vi "find_parameters.vi"(10 "script input":string) -> (0 "Parameter Array":string[](array[string]), 1 "plotnames":string, 2 "parameter string":string, 3 "command":string, 4 "number of parameters":u8)   [LabVIEW 2017]
doc: "splits the command, parameters and plotname from the input string.\n\ncommand syntax:\n\ncommand(param1;param2;...)->plot_name"
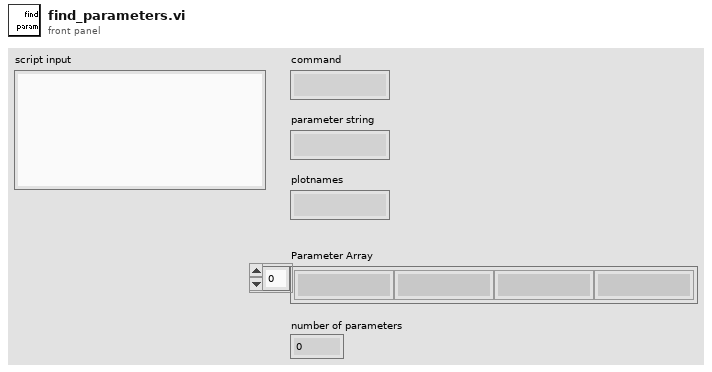
[diagram p1: front panel]
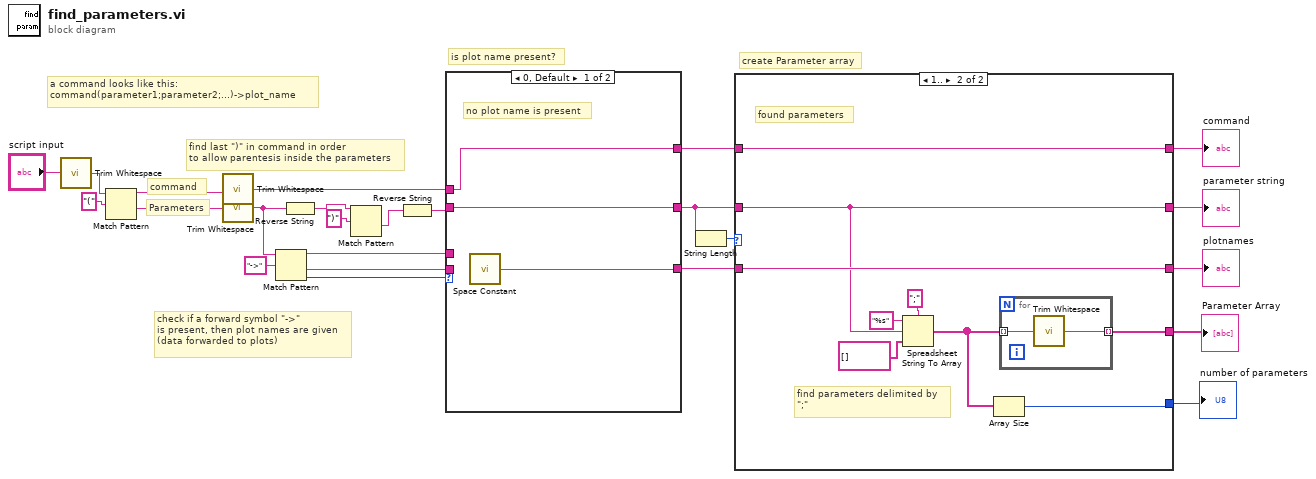
[diagram p0: block diagram]
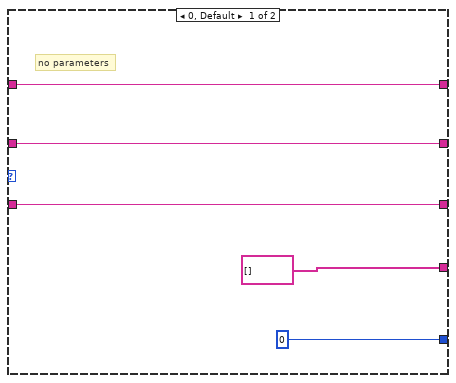
[diagram p2: hidden frame]
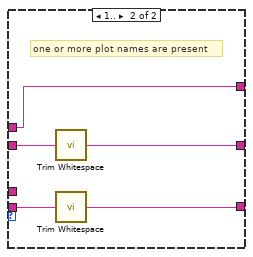
[diagram p3: hidden frame]
diagram:
  # "find last \")\" in command in order\nto allow parentesis inside the parameters"
  # "a command looks like this:\ncommand(parameter1;parameter2;...)->plot_name"
  # "is plot name present?"
  # "create Parameter array"
  # "Parameters"
  # "check if a forward symbol \"->\"\nis present, then plot names are given\n(data forwarded to plots)"
  # "command"
  n1 = call <vilib>:"Trim Whitespace.vi"("string"="script input") -> ("trimmed string"=w21:string)  [unwired: 1 in]
  n2 = Match Pattern(string=w21, regular expression="(") -> (before substring=w24:string, after substring=w23:string)  [unwired: 1 in, 2 out]
  n3 = call <vilib>:"Trim Whitespace.vi"("string"=w24) -> ("trimmed string"=w20:string)  [unwired: 1 in]
  n4 = call <vilib>:"Trim Whitespace.vi"("string"=w23) -> ("trimmed string"=w4:string)  [unwired: 1 in]
  n5 = Match Pattern(string=w4, regular expression="->") -> (before substring=w17:string, after substring=w16:string, offset past match=w18:i32)  [unwired: 1 in, 1 out]
  n6 = Reverse String(1:w4) -> (0:w3:string)
  n7 = Match Pattern(string=w3, regular expression=")") -> (after substring=w2:string)  [unwired: 1 in, 3 out]
  n8 = Reverse String(1:w2) -> (0:w1:string)
  n9 = case shown="0, Default" w18 {
    tunnel: w20 -> [w27 w32]
    tunnel: w1 -> [w25 w28]
    tunnel: [w27 w32] -> w13
    tunnel: [w25 w31] -> w10
    tunnel: [w26 w29] -> w12
    tunnel: w17 -> [_ _]
    tunnel: w16 -> [_ w30]
    frame 0, Default {
      # "no plot name is present"
      n10 = call <vilib>:"Space Constant.vi"() -> ("String"=w26:string)
    }
    frame 1.. {
      # "one or more plot names are present"
      n11 = call <vilib>:"Trim Whitespace.vi"("string"=w28) -> ("trimmed string"=w31:string)  [unwired: 1 in]
      n12 = call <vilib>:"Trim Whitespace.vi"("string"=w30) -> ("trimmed string"=w29:string)  [unwired: 1 in]
    }
  }
  n13 = String Length(string=w10) -> (length=w11:i32)
  n14 = case shown="1.." w11 {
    tunnel: w10 -> [w36 w41]
    tunnel: w13 -> [w37 w46]
    tunnel: w12 -> [w35 w45]
    tunnel: [w37 w46] -> w9
    tunnel: [w36 w41] -> w8
    tunnel: [w35 w45] -> w7
    tunnel: [u8 0 w40] -> w6
    tunnel: [string[] [] w38] -> w5
    frame 0, Default {
      # "no parameters"
    }
    frame 1.. {
      # "find parameters delimited by\n\";\""
      # "found parameters"
      n15 = Spreadsheet String To Array(delimiter (Tab)=";", format string="%s", spreadsheet string=w41, array type (2D Dbl)=string[] []) -> (array=w39:string[])
      n16 = Array Size(array=w39) -> (size(s)=w40:i32)
      n17 = for {
        tunnel: w39 -> [w48] mode=indexing
        tunnel: [w47] -> w38 mode=indexing
        n18 = call <vilib>:"Trim Whitespace.vi"("string"=w48) -> ("trimmed string"=w47:string)  [unwired: 1 in]
      }
    }
  }
  "command" <- w9
  "parameter string" <- w8
  "plotnames" <- w7
  "number of parameters" <- w6
  "Parameter Array" <- w5
